vi "UpdateQuery.vi"(8 "Error In":errorcluster, 10 "input cluster":T1, 11 "connection reference":T2) -> (0 "Error Out":errorcluster, 2 "Result_2D":string[][](array[string]), 4 "Result_1D":string[](array[string]), 5 "Element":string, 6 "Result_1D Row":string[](array[string]))   [LabVIEW 2020]
uses:
  <vilib>/addons/database/Connection.llb/Conn ObjectReference.ctl
  crearQry.dll
  <vilib>/addons/database/Connection.llb/Conn Execute.vi
  <vilib>/addons/database/Recordset.llb/Rec Fetch Recordset Data (R).vi
  <vilib>/addons/database/Recordset.llb/Rec Destroy - Connection.vi
  <vilib>/addons/database/_DB Variant To Data/Database Variant To Data.xnode
  <vilib>/addons/database/NI_Database_API.lvlib
panel:
  out "Records":i32
  out "sqlQry":string
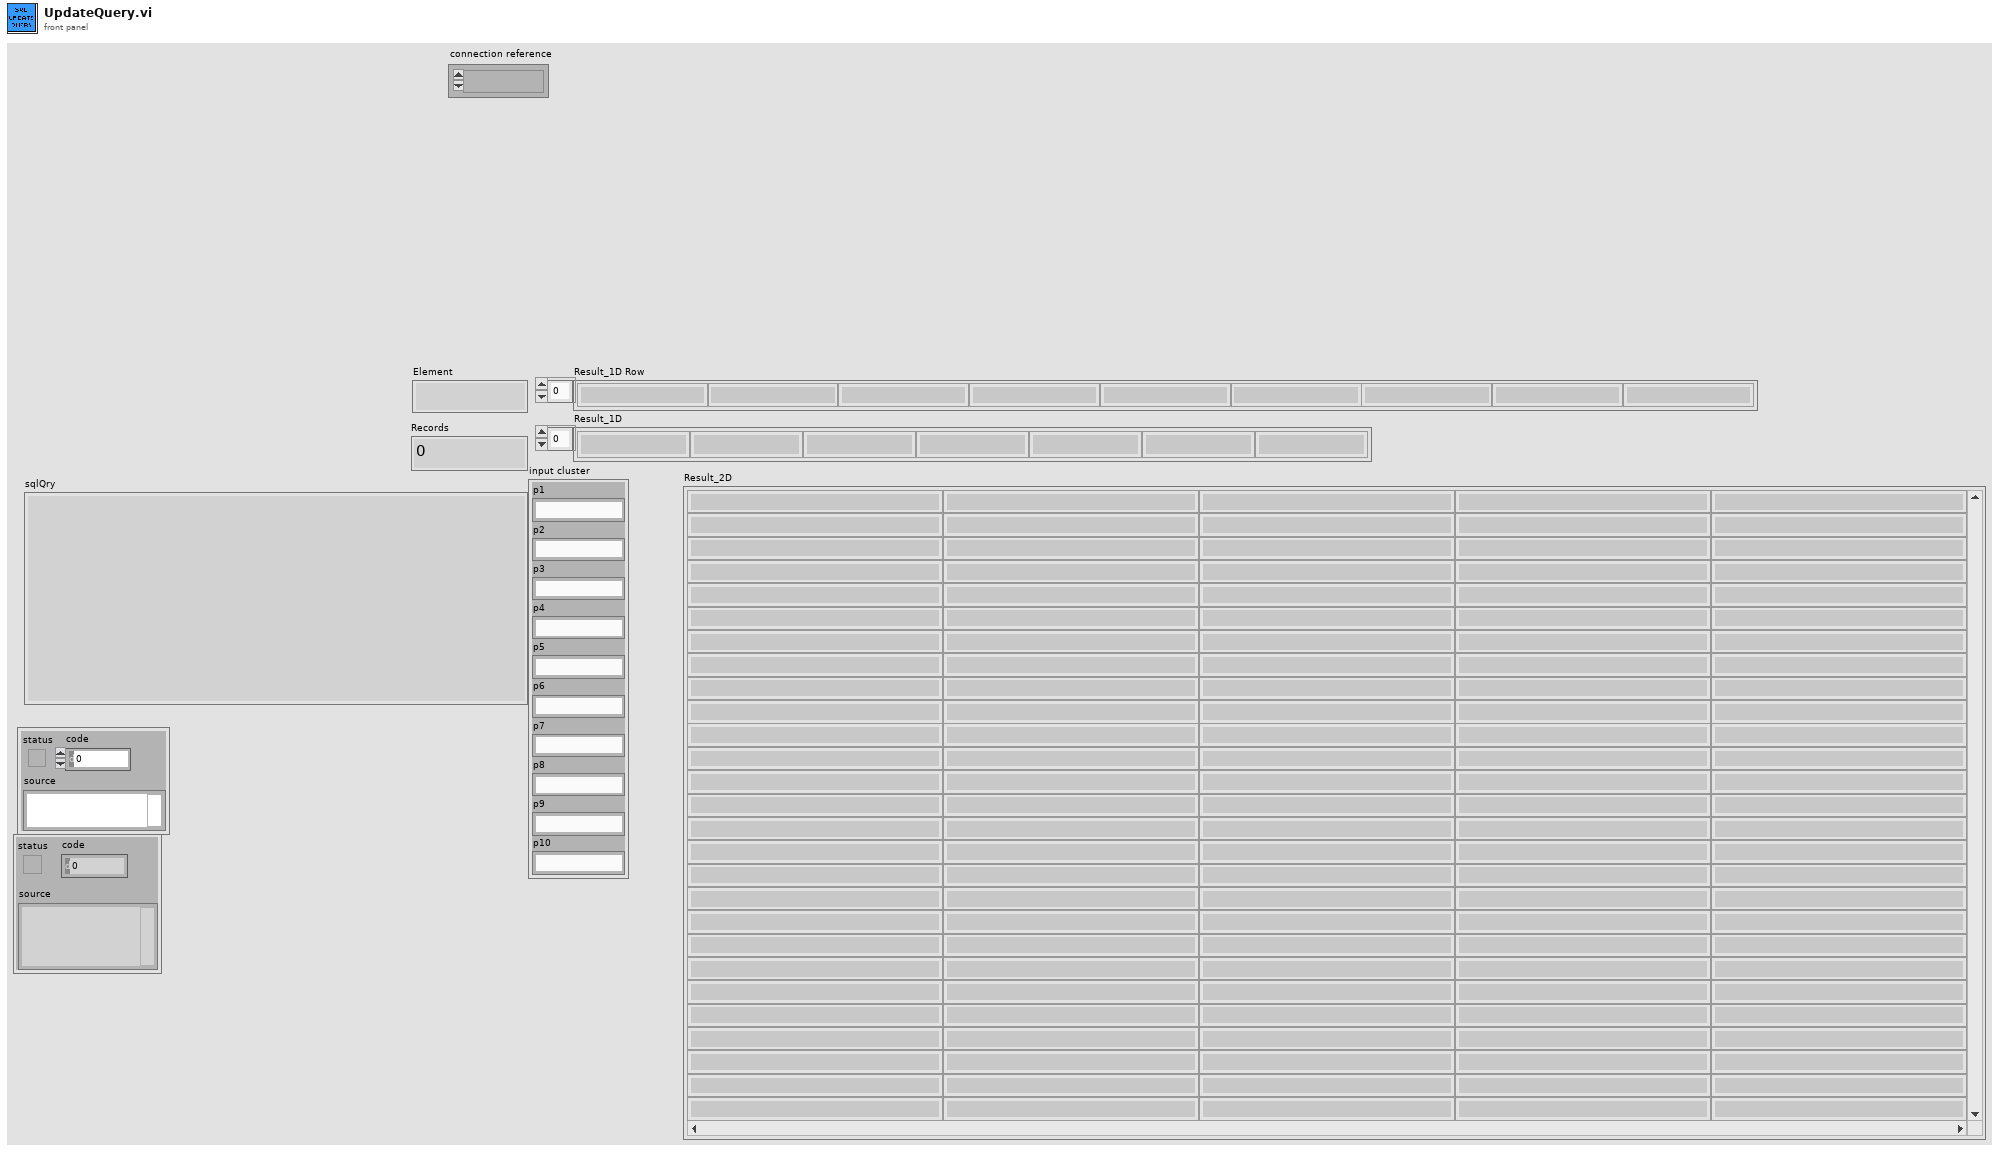
[diagram p1: front panel]
types:
  T1 = cluster{"p1":string, "p2":string, "p3":string, "p4":string, "p5":string, "p6":string, "p7":string, "p8":string, "p9":string, "p10":string}
  T2 = typedef "NI_Database_API.lvlib/Conn ObjectReference.ctl" = refnum<k1>
  T3 = typedef "NI_Database_API.lvlib/Rec ObjectReference.ctl" = refnum<k1>
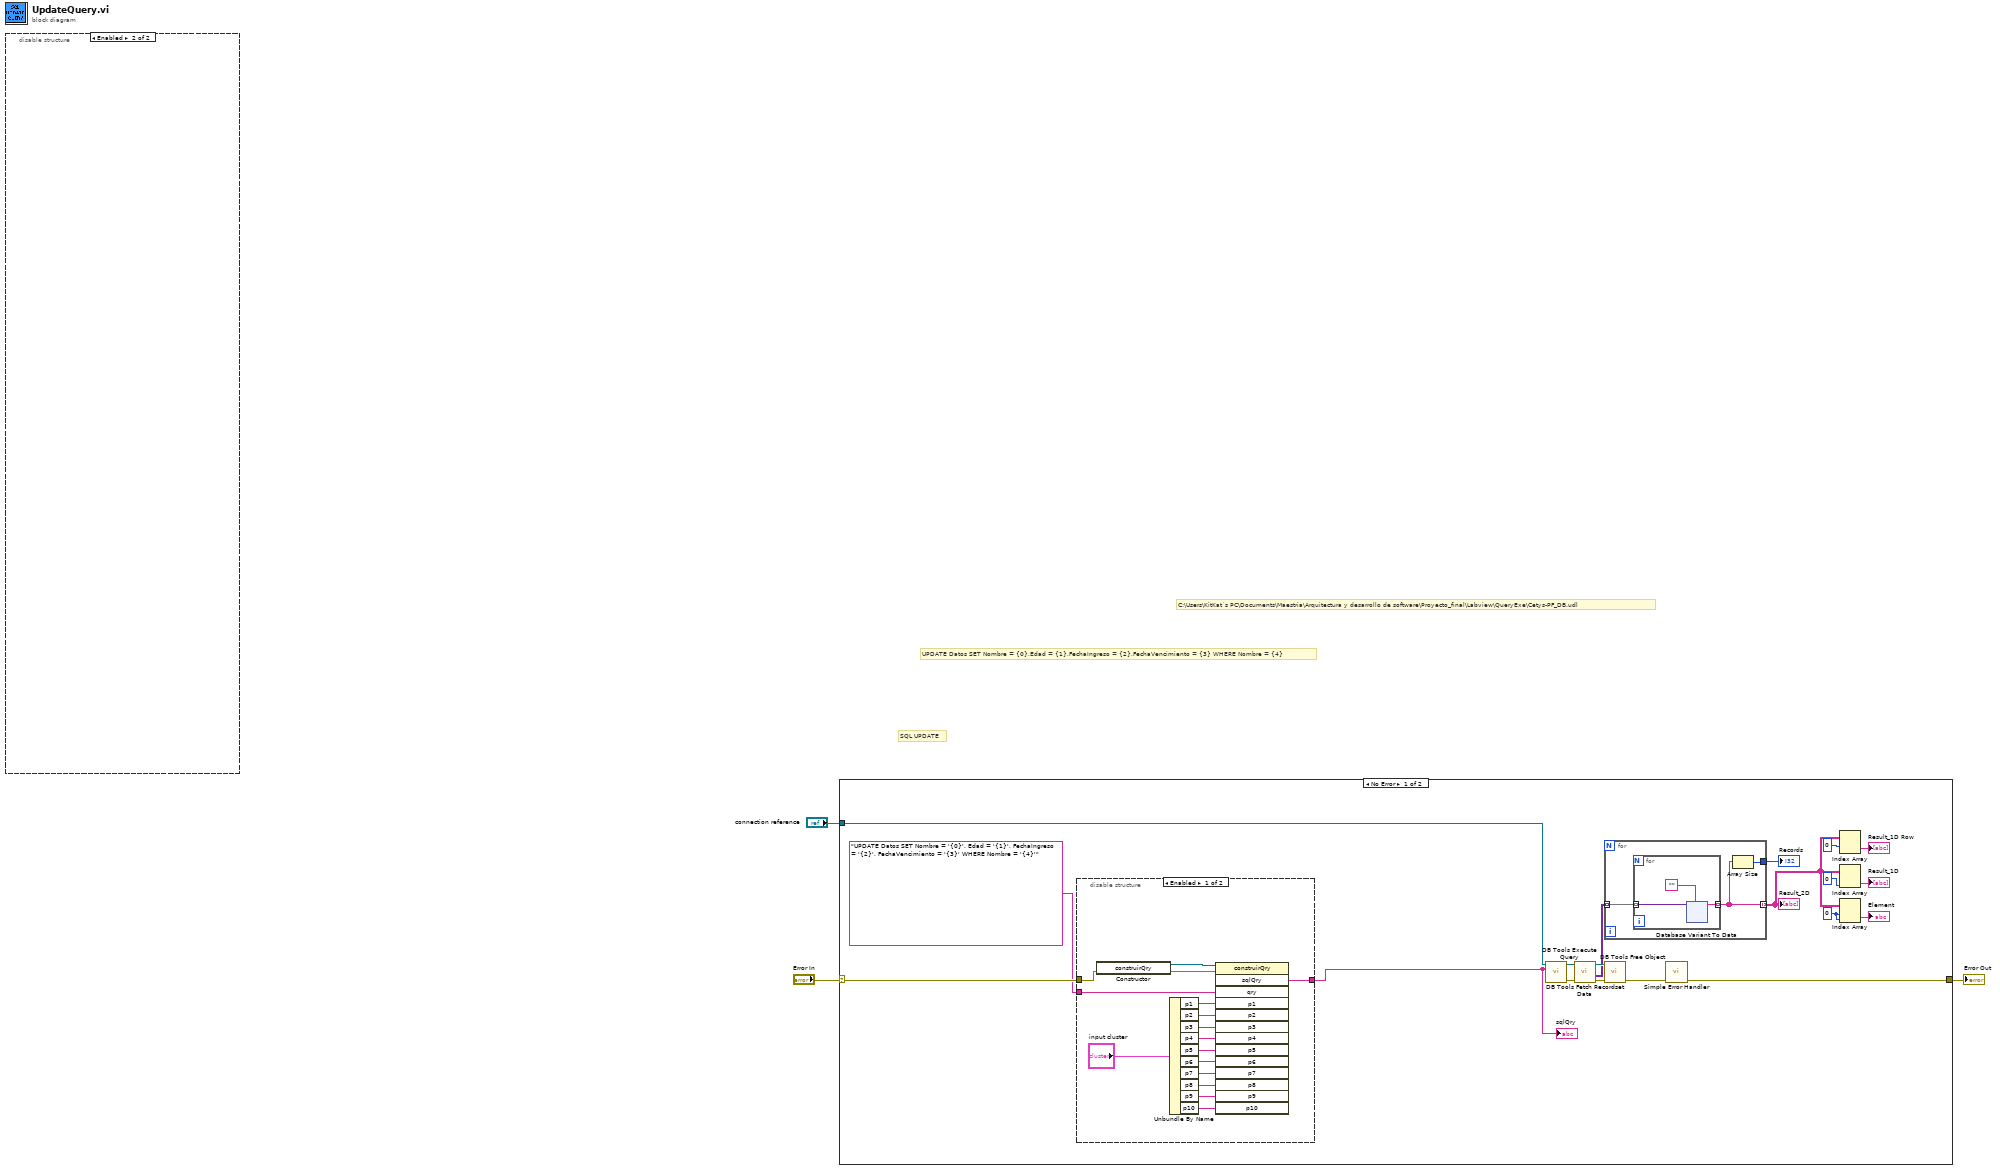
[diagram p0: block diagram]
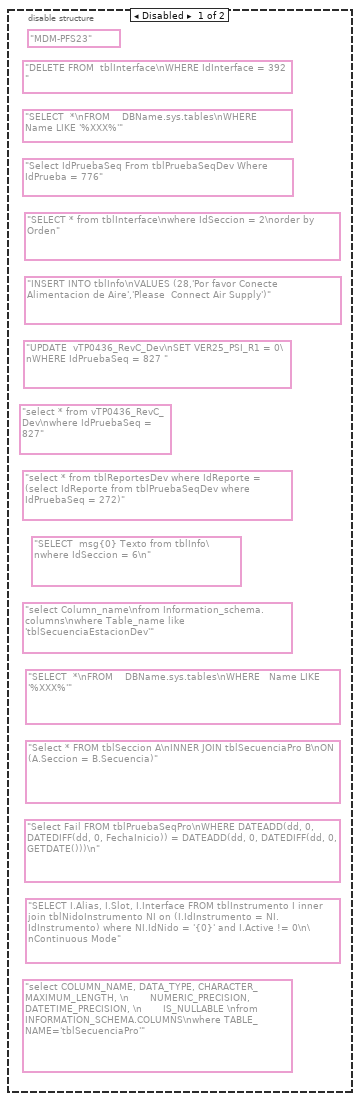
[diagram p4: hidden frame]
diagram:
  # "UPDATE Datos SET Nombre = {0},Edad = {1},FechaIngreso = {2},FechaVencimiento = {3} WHERE Nombre = {4}"
  # "SQL UPDATE"
  # "C:\\Users\\KitKat´s PC\\Documents\\Maestria\\Arquitectura y desarrollo de software\\Proyecto_final\\Labview\\QueryExe\\Cetys-PF_DB.udl"
  n1 = disable-structure shown="Enabled" {
    frame Disabled {
      (unwired) "SELECT  msg{0} Texto from tblInfo\nwhere IdSeccion = 6\n" ("qry")
      (unwired) "select * from vTP0436_RevC_Dev\nwhere IdPruebaSeq = 827" ("qry")
      (unwired) "MDM-PFS23" ("Nombre de PC")
      (unwired) "SELECT  *\nFROM    DBName.sys.tables\nWHERE   Name LIKE '%XXX%'" ("qry")
      (unwired) "Select Fail FROM tblPruebaSeqPro\nWHERE DATEADD(dd, 0, DATEDIFF(dd, 0, FechaInicio)) = DATEADD(dd, 0, DATEDIFF(dd, 0, GETDATE()))\n" ("qry")
      (unwired) "Select * FROM tblSeccion A\nINNER JOIN tblSecuenciaPro B\nON (A.Seccion = B.Secuencia)" ("qry")
      (unwired) "SELECT * from tblInterface\nwhere IdSeccion = 2\norder by Orden" ("qry")
      (unwired) "SELECT I.Alias, I.Slot, I.Interface FROM tblInstrumento I inner join tblNidoInstrumento NI on (I.IdInstrumento = NI.IdInstrumento) where NI.IdNido = '{0}' and I.Active != 0\n\nContinuous Mode" ("qry")
      (unwired) "select * from tblReportesDev where IdReporte = (select IdReporte from tblPruebaSeqDev where IdPruebaSeq = 272)" ("sqlQry")
      (unwired) "DELETE FROM  tblInterface\nWHERE IdInterface = 392 " ("qry")
      (unwired) "select COLUMN_NAME, DATA_TYPE, CHARACTER_MAXIMUM_LENGTH, \n       NUMERIC_PRECISION, DATETIME_PRECISION, \n       IS_NULLABLE \nfrom INFORMATION_SCHEMA.COLUMNS\nwhere TABLE_NAME='tblSecuenciaPro'" ("qry")
      (unwired) "SELECT  *\nFROM    DBName.sys.tables\nWHERE   Name LIKE '%XXX%'" ("qry")
      (unwired) "select Column_name\nfrom Information_schema.columns\nwhere Table_name like 'tblSecuenciaEstacionDev'" ("qry")
      (unwired) "Select IdPruebaSeq From tblPruebaSeqDev Where IdPrueba = 776" ("qry")
      (unwired) "UPDATE  vTP0436_RevC_Dev\nSET VER25_PSI_R1 = 0\nWHERE IdPruebaSeq = 827 " ("qry")
      (unwired) "INSERT INTO tblInfo\nVALUES (28,'Por favor Conecte Alimentacion de Aire','Please  Connect Air Supply')" ("qry")
    }
    frame Enabled {
    }
  }
  n2 = case shown="No Error" "Error In" {
    selector: "Error In" -> [w7 w78]
    tunnel: [w18 w78] -> w3
    tunnel: "connection reference" -> [w8 _]
    frame No Error {
      w15 = 0 ("index (row)")
      n3 = disable-structure shown="Enabled" {
        disable-tunnel: [w36 w39] -> w6
        disable-tunnel: w7 -> [w24 _]
        disable-tunnel: "UPDATE Datos SET Nombre = '{0}', Edad = '{1}', FechaIngreso = '{2}', FechaVencimiento = '{3}' WHERE Nombre = '{4}'" ("qry") -> [w23 w39]
        frame Enabled {
          n4 = constructor class="construirQry"(error in=w24) -> (reference out=w38:refnum<k24>, error out=w37:errorcluster)  [unwired: 2 in, 1 out]
          n5 = Unbundle By Name("input cluster") -> ("p1"=w35:string, "p2"=w34:string, "p3"=w33:string, "p4"=w32:string, "p5"=w31:string, "p6"=w30:string, "p7"=w29:string, "p8"=w28:string, "p9"=w27:string, "p10"=w26:string)
          n6 = invoke class="construirQry" method="sqlQry"(reference=w38, error in=w37, "qry"=w23, "p1"=w35, "p2"=w34, "p3"=w33, "p4"=w32, "p5"=w31, "p6"=w30, "p7"=w29, "p8"=w28, "p9"=w27, "p10"=w26) -> ("sqlQry"=w36:string)  [unwired: 1 in, 13 out]
        }
        frame Disabled {
        }
      }
      "sqlQry" <- w6
      n7 = call-poly <vilib>:"DB Tools Execute Query.vi"("SQL query"=w6, "connection reference"=w8) -> ("error out"=w21:errorcluster, "recordset reference"=w22:T3)  [unwired: 6 in]
      n8 = call-poly <vilib>:"DB Tools Fetch Recordset Data.vi"("error in (no error)"=w21, "recordset reference"=w22) -> ("error out"=w19:errorcluster, "recordset data"=w17:variant[][], "recordset reference out"=w20:T3)  [unwired: 3 in]
      n9 = for {
        tunnel: w17 -> [w42] mode=indexing
        tunnel: [w41] -> w11 mode=indexing
        tunnel: [w40] -> w16
        n10 = for {
          tunnel: w42 -> [w45] mode=indexing
          tunnel: [w44] -> w41 mode=indexing
          n11 = xnode "Database Variant To Data"("database variant"=w45, "type"="") -> ("data"=w44:string)  [unwired: 1 in, 1 out]
        }
        n12 = Array Size(array=w41) -> (size(s)=w40:i32)
      }
      "Result_2D" <- w11
      "Records" <- w16
      n13 = call-poly <vilib>:"DB Tools Free Object.vi"("error in (no error)"=w19, "recordset reference"=w20) -> ("error out"=w4:errorcluster)  [unwired: 8 in, 1 out]
      n14 = call <vilib>:"Simple Error Handler.vi"("error in (no error)"=w4) -> ("error out"=w18:errorcluster)  [unwired: 4 in, 4 out]
      n15 = Index Array(array=w11, index (row)=0 ("disabled index (col)")) -> (element=→"Result_1D Row":string[])  [unwired: 1 in]
      n16 = Index Array(array=w11, index (col)=0 ("disabled index (col)")) -> (element=→"Result_1D":string[])  [unwired: 1 in]
      n17 = Index Array(array=w11, index (row)=w15, index (col)=w15) -> (element=→"Element":string)
    }
    frame Error {
    }
  }
  "Error Out" <- w3
